vi "Big_LED_control.vi"() -> ()   [LabVIEW 2018]
uses:
  <instrlib>/niDCPower/nidcpower.llb/niDCPower Source Mode.ctl
  <instrlib>/niDCPower/nidcpower.llb/niDCPower Output Function.ctl
  AT lib/AmateurStepperMotor.dll
  <instrlib>/niDMM/nidmm.llb/niDMM Function.ctl
  <instrlib>/niDMM/nidmm.llb/niDMM Resolution in Digits.ctl
  <vilib>/Instr/_visa.llb/VISA Configure Serial Port (Instr).vi
  <instrlib>/niDMM/nidmm.llb/niDMM Configure Measurement Digits.vi
panel:
  out "voltmes_I_LED, V":dbl=-0.00011794146773492402 caption="measurement" format="%_6g"
  out "curmes_I_LED, A":dbl=4.978853713564661e-05 caption="measurement" format="%_6g"
  out "curmes_V_MB, A":dbl=4.978853713564661e-05 caption="measurement" format="%_6g"
  out "voltmes_V_MB, V":dbl=-0.00019003121552656476 caption="measurement" format="%_6g"
  in  "Tab Control 2":enum32{"Шаговик и офир", "Служебная область"}(tab)
  in  "milliseconds to wait":u32=1000
  in  "Go To":dbl
  out "Ophir 1 Char":dbl(graph)=0.02
  in  "DecelerationTime, s":dbl=0.3
  in  "AccelerationTime, s":dbl=0.3
  in  "HoldOn":bool
  in  "Ophir 1 units":string(combo)="1000" caption="Units"
  out "Ophir 1 Over Range":bool caption="Over Range"
  out "Ophir 1 Optical Power":dbl=0.02 caption="Power" format="%#_4g"
  out "Ophir 1 MAX":dbl=0.030000000000000002 caption="MAX" format="%#_5g"
  in  "Ophir 1 Clear":bool caption="Clear"
  in  "StepMultiplicationFactor":dbl=50.0
  in  "StepDivisor":i32(ring)=8 items=["D1"=1, "D2"=2, "D4"=4, "D8"=8, "D16"=16, "D32"=32]
  in  "Speed":dbl=250.0
  in  "Погнали!":bool=TRUE
  in  "Стоп GoTo":bool
  out "Готово":bool
  out "Position":dbl
  in  "Ophir 1 Info":u16(ring)=1 caption="Info" items=["Device : JUNO; s/n:903793", "Head : PD300R-3W   ; s/n:779628"]
  in  "new pos":dbl
  in  "set pos":bool
  out "Device Response":string="*\n"
  in  "Ophir 1 usb channel":i16 caption="usb channel"
  out "Ophir 1 dup Visa Session":refnum<visa-resource-name>="USB0::0x0BD3::0x0777::NI-VISA-60004::RAW" caption="dup Visa Session"
  in  "Ophir 1 Baud Rate (3:9600)":i16(ring)=3 caption="Baud Rate (3:9600)" items=["300", "1200", "4800", "9600", "19200", "38400"]
  out "Ophir 1 Real Optical Power":dbl=2e-05 format="%.6e"
  in  "Ophir 1 GPIB Address (10)":string="10" caption="GPIB Address (10)"
  in  "Ophir 1 Port Number (default 2)":i16=1 caption="Port Number (default 2)" min=0 max=20
  in  "Ophir 1 Select Communication Protocol":u16(ring) caption="Select Communication Protocol" items=["USB", "RS232", "GPIB"]
  out "Ophir 1 error out":errorcluster caption="error out"
  in  "Ophir 1 error in (no error)":errorcluster caption="error in (no error)"
  in  "Ophir 1 Wait":u32=100 caption="Wait"
  out "IsOpen":bool=TRUE
  out "Ophir 1 Initialization":bool=TRUE caption="Initialization"
  in  "Tab Control":T1(tab)
  in  "POWER":bool
  in  "Стоп":bool=TRUE
  in  "Resource Name":refnum<k15>="PXI1Slot2" caption="Источник питания"
  in  "Амперметр":refnum<k15>="PXI1Slot4" caption="NI DMM 1"
  in  "V_MB, V":dbl=2.0 caption="voltage level" format="%_6p"
  in  "curlim_V_MB, A":dbl=0.3 caption="current limit" format="%_6p"
  out "chart_0":dbl(graph)=-0.00019003121552656476 caption="Waveform Chart 5"
  in  "voltlim_I_LED, V":dbl=2.0 caption="current limit" min=0.01 format="%_6p"
  in  "I_LED, A":dbl=0.005 caption="voltage level" format="%_6p"
  out "chart_1":dbl(graph)=-0.00011794146773492402 caption="Waveform Chart 5"
  out "Current Char":dbl(graph)=0.004513189196586609
  in  "Arduino":refnum<visa-resource-name>="COM14"
  in  "Сегменты":bool[](array[boolean])=[FALSE, FALSE, FALSE, FALSE, FALSE, FALSE, FALSE, FALSE, FALSE, FALSE, FALSE, FALSE, FALSE, FALSE, FALSE, FALSE, FALSE, FALSE]
  in  "Вольтметр":refnum<k15>="PXI1Slot5" caption="NI DMM 1"
  out "Voltage Char":dbl(graph)=0.015767553821206093
  in  "Port Name":string="COM4" caption="Порт шаговика"
  in  "wave_lenght":string="600"
  in  "Промер":bool caption="Промер сегмента"
  in  "NI DMM 1 Voltage Range 4":string(combo)="-1" caption="Range"
  in  "NI DMM 1 units 4":string(combo)="1" caption="Units"
  out "Voltage":dbl=0.015767553821206093 format="%_6g"
  in  "NI DMM 1 Current Range 3":string(combo)="1" caption="Range"
  in  "NI DMM 1 units 3":string(combo)="1000" caption="Units"
  out "Current":dbl=0.004513189196586609 format="%_6g"
  out "element":dbl
  out "element 2":dbl
  out "Разряд":dbl
  out "+/-":bool
  out "Power off":bool=TRUE
  in  "Command":string="Cathode"
  in  "Записать":bool
  out "measure output file refnum":refnum<file>
  out "Voltage, V":dbl=0.015767553821206093 caption="Measurement" format="%.5f"
  out "Current, A":dbl=4.513189196586609e-06 caption="Measurement" format="%.5f"
  out "Тип индикатора":string="Cathode"
  out "chart_2":dbl(graph)=-0.000179732680132088
  in  "V_RES, V":dbl caption="voltage level" format="%_6p"
  out "curmes_V_RES, A":dbl=5.996099535583298e-05 caption="measurement" format="%_6g"
  in  "curlim_V_RES, A":dbl=0.1 caption="current limit" min=0.01 format="%_6p"
  in  "measure path":path=path "D:/NI LabVIEW/MultiOpto/MultiOpto_1.2/Logs/SEL"
  out "Enum":enum16{"Exit", "4", "Промер", "2", "1"}(ring)
  out "№ об-ца":dbl=1.0
  out "Темп-ра":dbl=1.0
  out "Сегмент":string
  out "voltmes_V_RES, V":dbl=-0.000179732680132088 caption="measurement" format="%_6g"
  in  "current level range":dbl=0.001 format="%#.6p"
  # "Шаговик"
  # "Офир"
  # "Шаговик"
  # "Офир"
  # "position - это значение абсолютное"
  # "j"
  # "c"
  # "d"
  # "e"
  # "g"
  # "h"
  # "a"
  # "b"
  # "f"
  # "k"
  # "L"
  # "m"
  # "n"
  # "p"
  # "dp"
  # "all"
  # "V_MB 5 В\nогрничение 300 м\n\nV_LED 2,1 В\nограничение 200 м"
  # "единицы мА\nrange 1 А"
  # "1. каждый сегмент включаем по отдельности, резистором постраиваем ток до 10 мА\n2. напряжение V_LED при этом не меняется\n3. в такоом положении промеряем сегменты по отдельности\n4. для промера всего индикатора сразу подстраиваем напряжение при неизменном положении резисторов\n5. ток всех индикаторов = ток одного сегмента (10 мА) * число сегментов (15)\n6. добиваемся этого увеличением V_LED"
  # "единицы В\nrange AUTO"
  # "регклировка суммарного тока через индикатор"
  # "24.063\n\n     I          U\n20 мА  1.3 В\n20 мА  1.4 В\n 7 мА   1.15 В"
  # "24.064\n\n     I          U\n10 мА  2 В\n10 мА  2.15 В\n 7 мА   1.9 В"
  # "автоматизировать подбор напряжения по известному максимальному напряжению и току. ОС по току сегмента"
  # "Р1:  +25°C\nР2:  - 60°C\nР3:  +85°C"
  # "регулировать ток в зависимости от температуры.\nс ростом температуры растет ток.\nпид-регулятор??"
  # "0. ввести номер образца\n1. включить нужный сегмент\n2. ввести его в поле справа\n3. вести температуру в поле слева\n4. нажать кнопку \"промер сегмента\""
  # "\"опрашивать кнопки не чаще, чем раз в секунду. сейчас кликать можно чаще, они загорятся, но ничего не произойдет\""
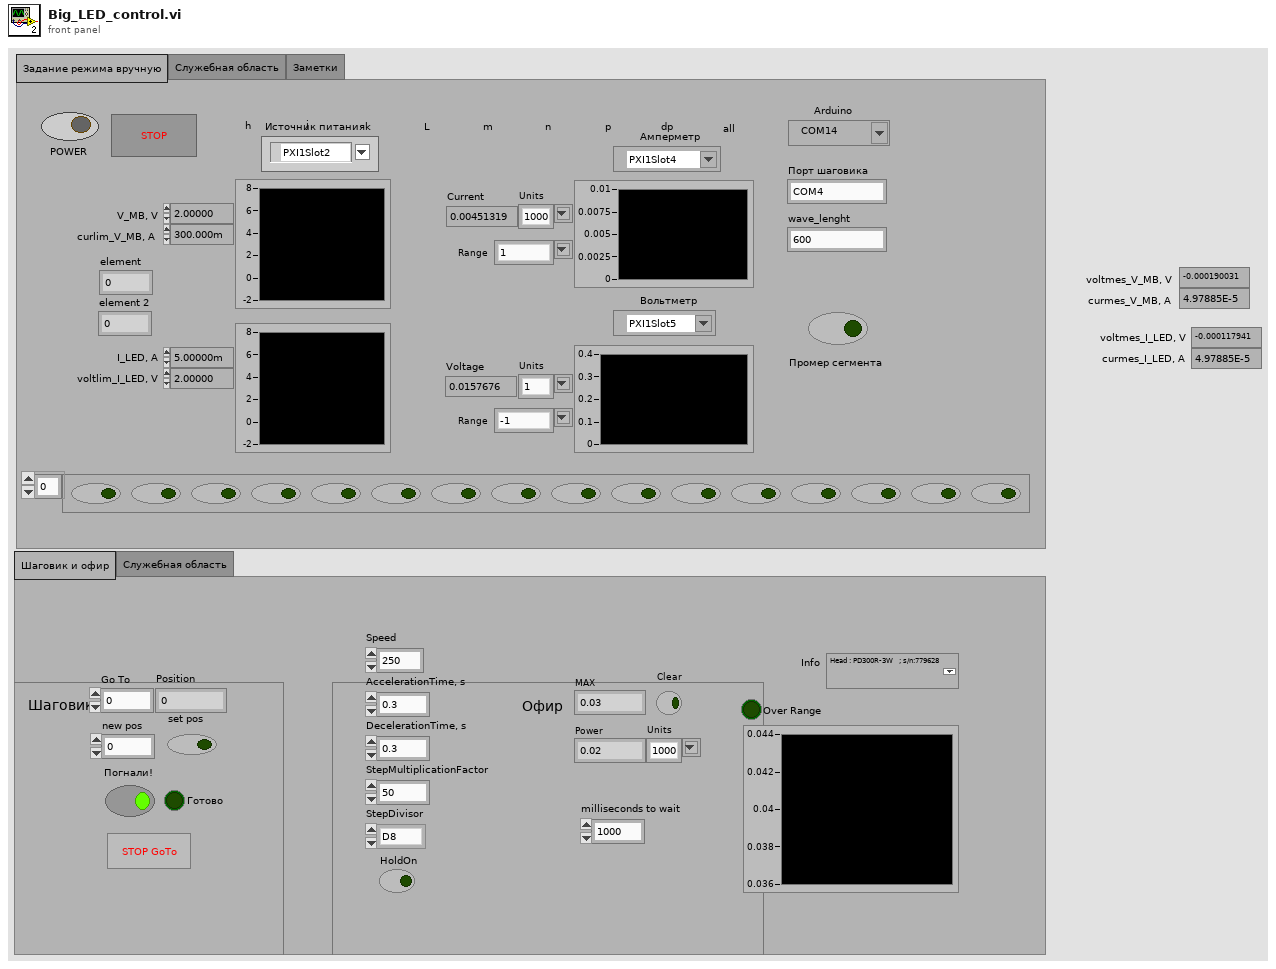
[diagram p1: front panel]
types:
  T1 = enum32{"Задание режима вручную", "Служебная область", "Заметки"}
  T2 = enum16{"open", "replace", "create", "open or create", "replace or create", "replace or create with confirmation"}
  T3 = typedef "niDCPower Output Function.ctl" = i32
  T4 = typedef "niDCPower Source Mode.ctl" = i32
  T5 = typedef "niDMM Function.ctl" = enum16{"DC Volts", "AC Volts", "DC Current", "AC Current", "2-wire Resistance", "4-wire Resistance", "Diode", "Frequency", "Period", "AC Volts DC Coupled", "Capacitance", "Inductance", "Temperature"}
  T6 = typedef "niDMM Resolution in Digits.ctl" = dbl
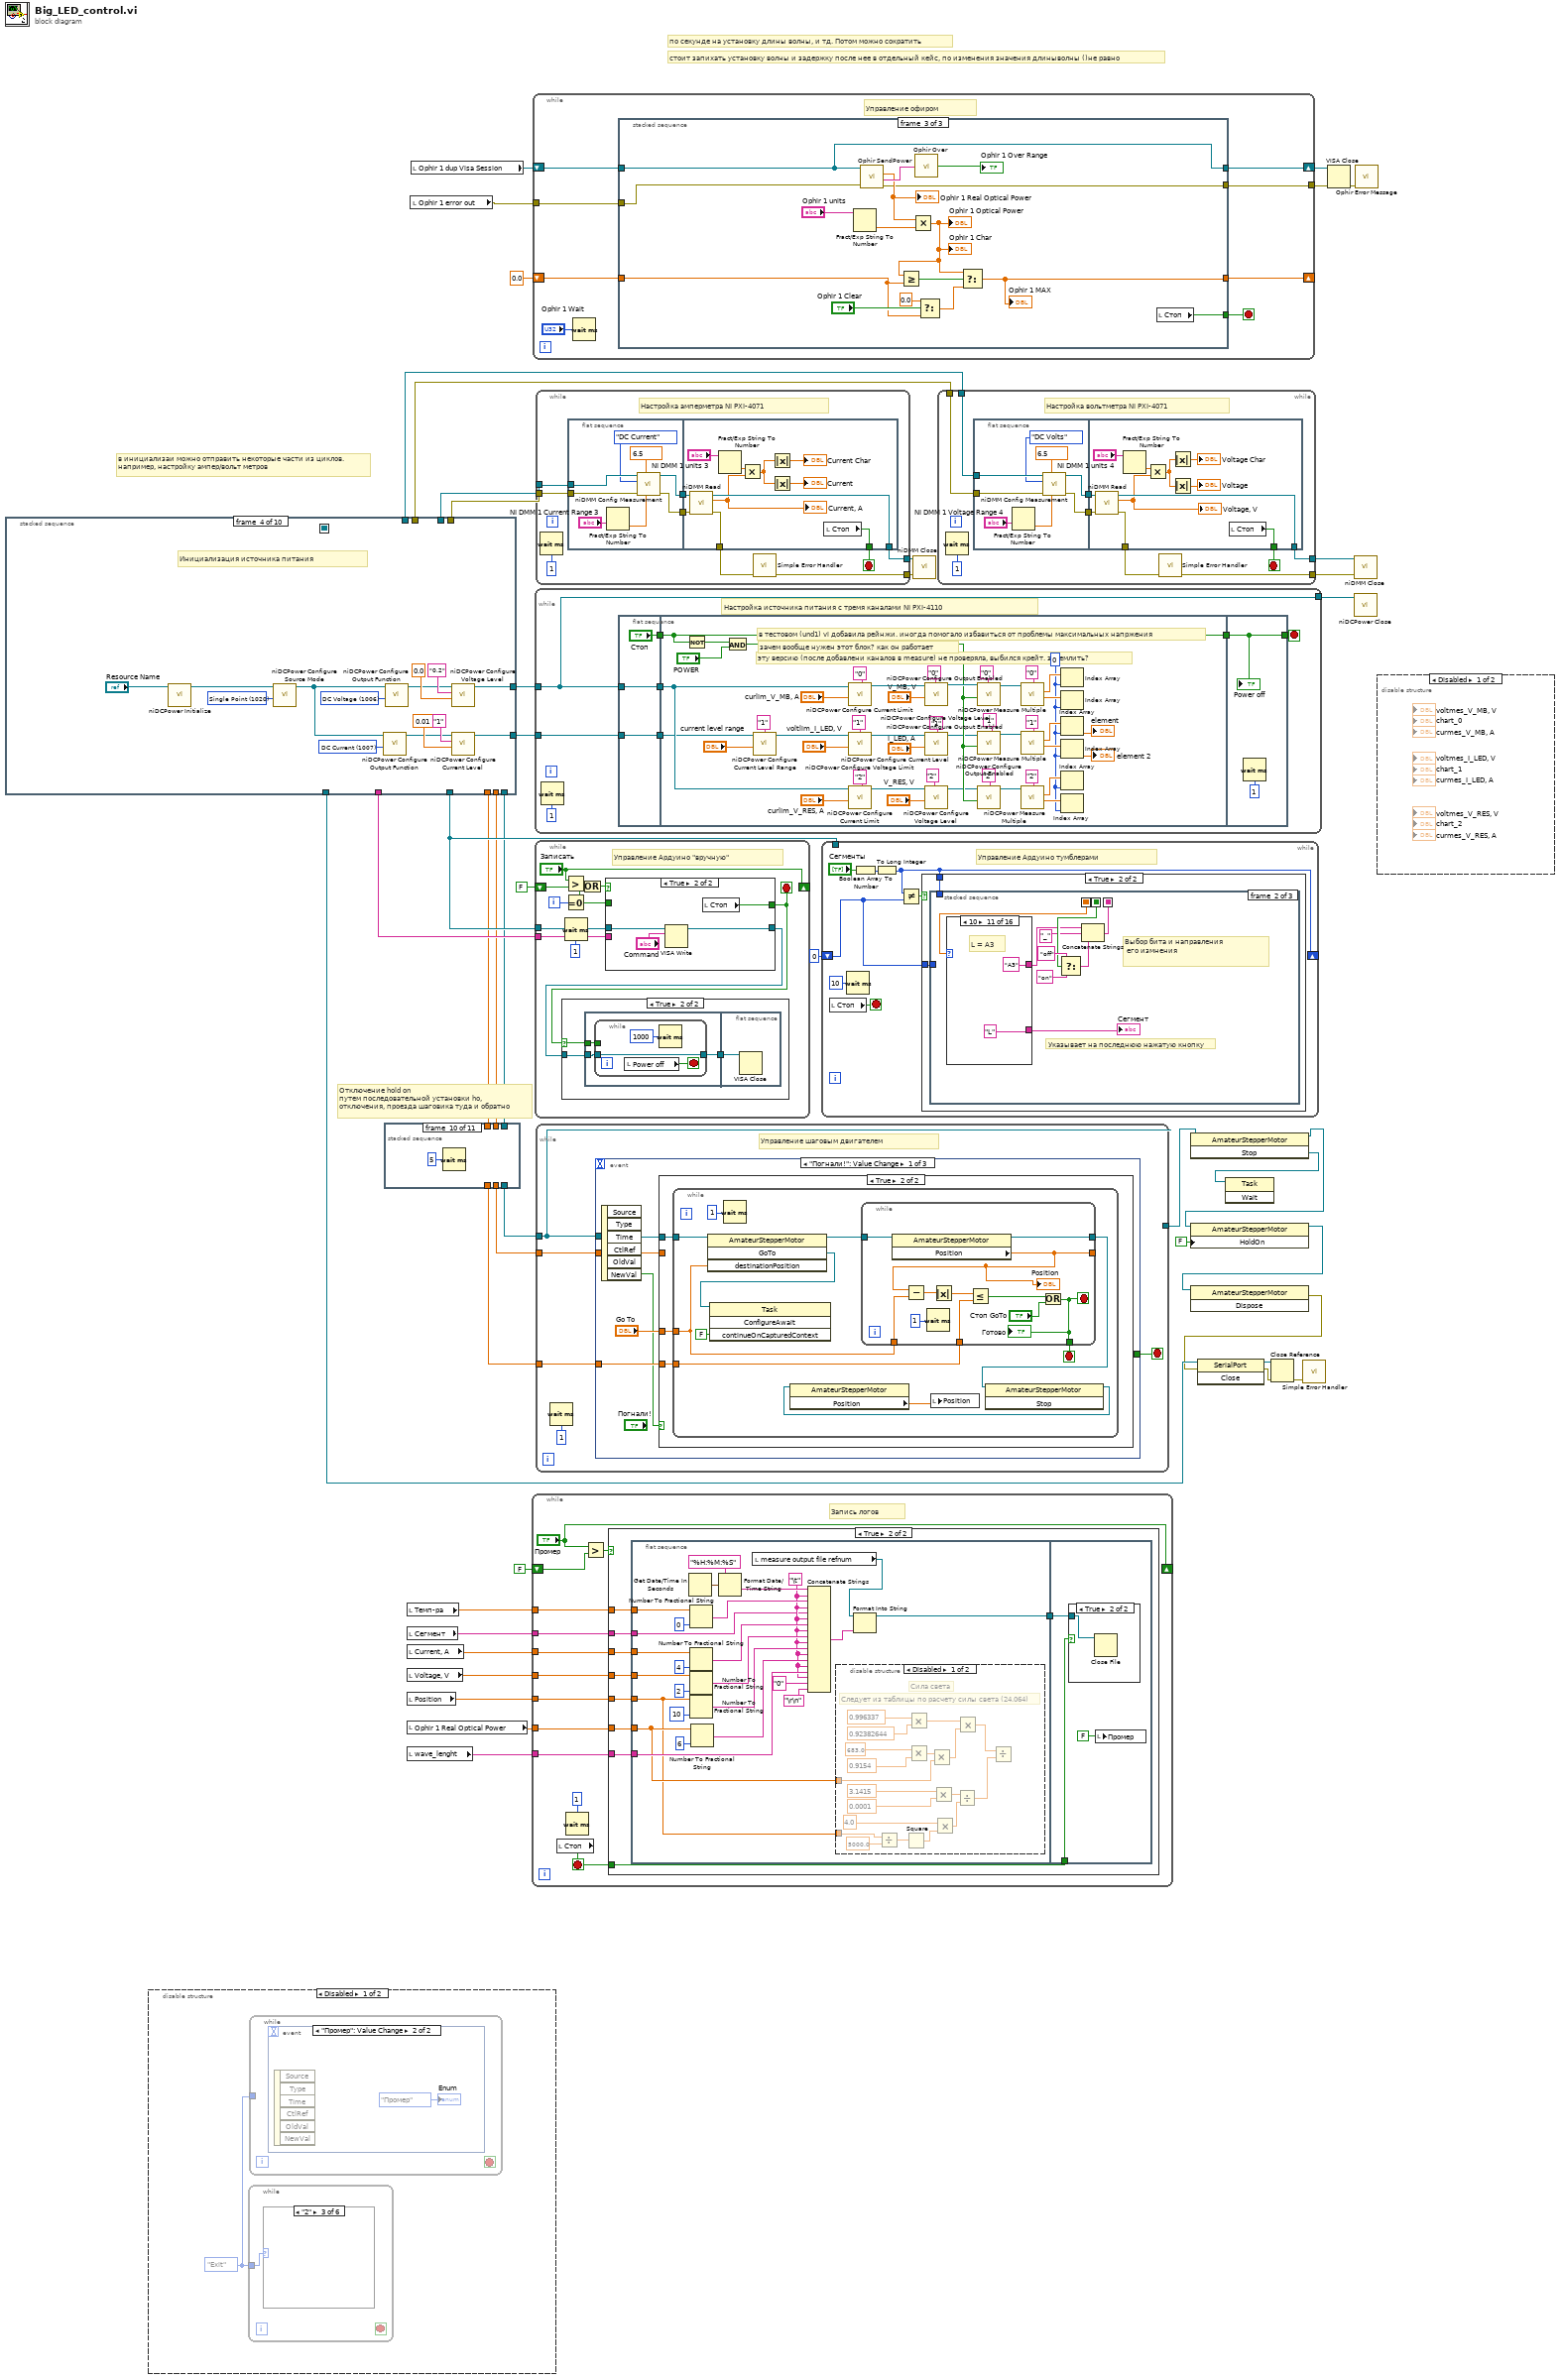
[diagram p0: block diagram]
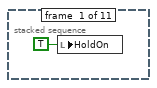
[diagram p3: hidden frame]
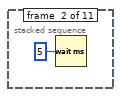
[diagram p4: hidden frame]
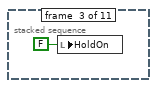
[diagram p5: hidden frame]
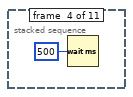
[diagram p6: hidden frame]
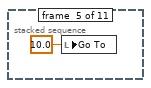
[diagram p7: hidden frame]
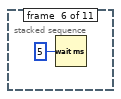
[diagram p8: hidden frame]
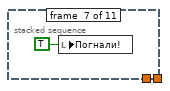
[diagram p9: hidden frame]
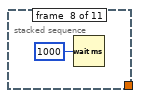
[diagram p10: hidden frame]
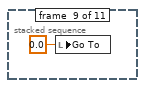
[diagram p11: hidden frame]
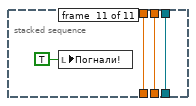
[diagram p12: hidden frame]
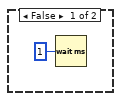
[diagram p13: hidden frame]
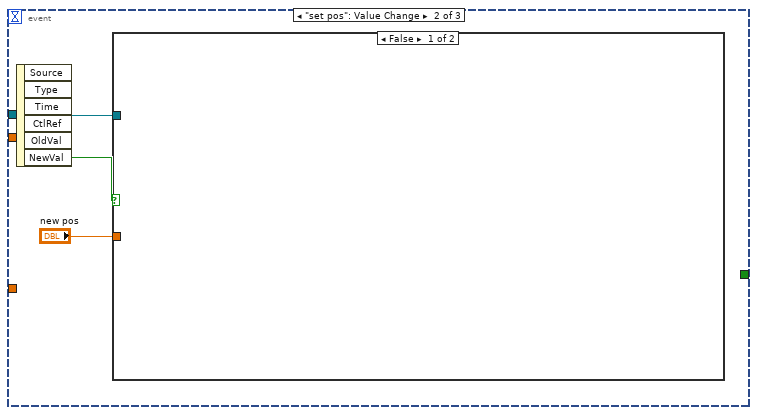
[diagram p14: hidden frame]
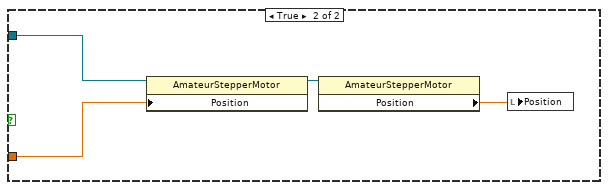
[diagram p15: hidden frame]
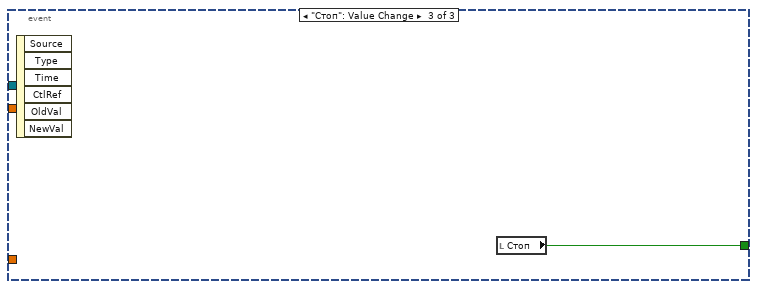
[diagram p16: hidden frame]
diagram:
  # "Отключение hold on\nпутем последовательной установки ho, \nотключения, проезда шаговика туда и обратно"
  # "в инициализаи можно отправить некоторые части из циклов.\nнапример, настройку ампер/вольт метров"
  # "стоит запихать установку волны и задержку после нее в отдельный кейс, по изменения значения длиныволны ()не равно"
  # "по секунде на установку длины волны, и тд. Потом можно сократить"
  n1 = stacked-sequence {
    seq-local: [_ _ _ _ _ _ w108 _ _ _] -> [_ _ _ _ _ _ _ w117 _ _]
    tunnel: [_ _ _ w74 _ _ _ _ _ _] -> w33
    tunnel: [_ w57 _ _ _ _ _ _ _ _] -> w45
    tunnel: [_ w56 _ _ _ _ _ _ _ _] -> w44
    tunnel: [_ _ _ _ w75 _ _ _ _ _] -> w41
    tunnel: [_ _ _ _ _ _ _ _ _ w155] -> w40
    tunnel: [_ _ w60 _ _ _ _ _ _ _] -> w39
    tunnel: [_ _ w59 _ _ _ _ _ _ _] -> w38
    tunnel: [_ _ _ _ _ _ _ w120 _ _] -> w1
    tunnel: [_ _ _ _ _ _ _ w118 _ _] -> w4
    tunnel: [_ _ _ _ _ _ _ w119 _ _] -> w6
    tunnel: [_ _ _ _ _ _ w98 _ _ _] -> w27
    tunnel: [_ _ _ w68 _ _ _ _ _ _] -> w10
    frame #0 {
      w51 = 0.0 ("currentmes_2")
      w52 = FALSE ("Стоп")
      # "ch 1"
      # "Обнуление переменных"
      n2 = local write "POWER"(w52) -> ()
      n3 = local write "Стоп"(w52) -> ()
      n4 = local write "+/-"(w52) -> ()
      n5 = local write "Погнали!"(w52) -> ()
      n6 = local write "Готово"(w52) -> ()
      n7 = local write "Стоп GoTo"(w52) -> ()
      n8 = local write "Speed"(250.0 ("Speed")) -> ()
      n9 = local write "StepMultiplicationFactor"(50.0 ("StepMultiplicationFactor")) -> ()
      n10 = local write "AccelerationTime, s"(0.3 ("AccelerationTime, s")) -> ()
      n11 = local write "DecelerationTime, s"(0.3 ("DecelerationTime, s")) -> ()
      n12 = local write "Go To"(w51) -> ()
      n13 = local write "curmes_V_MB, A"(w51) -> ()
      n14 = local write "curmes_V_RES, A"(w51) -> ()
      n15 = local write "Current"(w51) -> ()
      n16 = local write "Разряд"(w51) -> ()
      n17 = local write "voltmes_I_LED, V"(w51) -> ()
      n18 = local write "Сегменты"(bool[] [FALSE, FALSE, FALSE, FALSE, FALSE, FALSE, FALSE, FALSE, FALSE, FALSE, FALSE, FALSE, FALSE, FALSE, FALSE, FALSE, FALSE, FALSE] ("Сегменты")) -> ()
      n19 = local write "current level range"(0.001 ("current level range")) -> ()
      n20 = local write "Command"("zero" ("Command 2")) -> ()
    }
    frame #1 {
      # "Инициализация амперметра"
      n21 = call <instrlib>:"niDMM Initialize.vi"("Instrument Descriptor"="Амперметр") -> ("error out"=w57:errorcluster, "instrument handle out"=w56:refnum<k15>)  [unwired: 9 in]
    }
    frame #2 {
      # "Инициализация вольтметра"
      n22 = call <instrlib>:"niDMM Initialize.vi"("Instrument Descriptor"="Вольтметр") -> ("error out"=w59:errorcluster, "instrument handle out"=w60:refnum<k15>)  [unwired: 9 in]
    }
    frame #3 {
      w61 = T3 1007 items=["DC Voltage"=1006, "DC Current"=1007, "Pulse Voltage"=1049, "Pulse Current"=1050] ("output function")
      w62 = T3 1006 items=["DC Voltage"=1006, "DC Current"=1007, "Pulse Voltage"=1049, "Pulse Current"=1050] ("output function")
      w66 = T4 1020 items=["Single Point"=1020, "Sequence"=1021] ("source mode")
      # "Инициализация источника питания"
      n23 = call <instrlib>:"niDCPower Initialize.vi"("resource name"="Resource Name") -> ("instrument handle out"=w67:refnum<k15>)  [unwired: 3 in, 7 out]
      n24 = call <instrlib>:"niDCPower Configure Source Mode.vi"("source mode"=w66, "instrument handle"=w67) -> ("instrument handle out"=w65:refnum<k15>)  [unwired: 1 in, 8 out]
      n25 = call <instrlib>:"niDCPower Configure Output Function.vi"("output function"=w61, "instrument handle"=w65) -> ("instrument handle out"=w63:refnum<k15>)  [unwired: 8 in, 1 out]
      n26 = call <instrlib>:"niDCPower Configure Output Function.vi"("output function"=w62, "instrument handle"=w65) -> ("instrument handle out"=w64:refnum<k15>)  [unwired: 8 in, 1 out]
      n27 = call <instrlib>:"niDCPower Configure Voltage Level.vi"("voltage level"=0.0, "channel name"="0,2", "instrument handle"=w64) -> ("instrument handle out"=w74:refnum<k15>)  [unwired: 7 in, 1 out]
      n28 = call <instrlib>:"niDCPower Configure Current Level.vi"("current level"=0.01, "channel name"="1", "instrument handle"=w63) -> ("instrument handle out"=w68:refnum<k15>)  [unwired: 7 in, 1 out]
    }
    frame #4 {
      # "Инициализация Ардуино"
      n29 = call-poly "VISA Configure Serial Port"("VISA resource name"="Arduino", "baud rate (9600)"=u32 9600) -> ("VISA resource name out"=w75:refnum<visa-resource-name>)  [unwired: 12 in, 1 out]
    }
    frame #5 {
      # "Инициализация офира"
      n30 = call "Ophir InitCom.vi"("GPIB Address (default 10)"="Ophir 1 GPIB Address (10)", "Communication (default USB 0)"="Ophir 1 Select Communication Protocol", "USB Channel number (default 0)"="Ophir 1 usb channel", "Port Number (default 2)"="Ophir 1 Port Number (default 2)", "error in (no error)"="Ophir 1 error in (no error)", "Baud Rate (3:9600)"="Ophir 1 Baud Rate (3:9600)") -> ("dup Visa Session"=w84:refnum<visa-resource-name>, "error out"=w83:errorcluster)  [unwired: 1 out]
      n31 = call "Ophir InstrInfo.vi"("Visa Session"=w84, "error in (no error)"=w83) -> ("dup Visa Session"=w96:refnum<visa-resource-name>, "Instrument Info"=w78:string, "error out"=w94:errorcluster)
      n32 = call "Ophir HeadInfo.vi"("Visa Session"=w96, "error in (no error)"=w94) -> ("error out"=w93:errorcluster, "dup Visa Session"=w95:refnum<visa-resource-name>, "Head Info"=w92:string)  [unwired: 6 out]
      n33 = call "Ophir InfoStrings.vi"("error in (no error)"=w93, "Head Info"=w92, "Instrument Info"=w78) -> ("error out"=w91:errorcluster, "Strings Array"=w90:string[])
      n34 = property on="Ophir 1 Info" class="Ring (strict)"("Strings []"=w90) -> ()  [unwired: 2 in, 2 out]
      n35 = call "Ophir ConfigDevice.vi"("Visa Session"=w95, "Measure Choice (0:Power)"=u16 0, "error in (no error)"=w91) -> ("dup Visa Session"=→"Ophir 1 dup Visa Session":refnum<visa-resource-name>, "OK ?"=→"Ophir 1 Initialization":bool, "error out"=→"Ophir 1 error out":errorcluster)  [unwired: 1 out]
    }
    frame #6 {
      w102 = 100 ("WriteTimeout")
      w107 = 1 items=["None", "One", "Two", "OnePointFive"] ("stopBits")
      w104 = 0 items=["None", "Odd", "Even", "Mark", "Space"] ("parity")
      # "убрали открытие порта. шаговик его и так сам откроет"
      # "Инициализация шаговика ч.1"
      n36 = constructor class="SerialPort"("portName"="Port Name", "baudRate"=57600, "parity"=w104, "dataBits"=8, "stopBits"=w107) -> (reference out=w101:refnum<k24>, error out=w100:errorcluster)  [unwired: 3 in, 6 out]
      n37 = property class="SerialPort"(reference=w101, error in=w100, "WriteTimeout"=w102, "ReadTimeout"=w102) -> (reference out=w98:refnum<k24>)  [unwired: 1 out]
      n38 = constructor class="AmateurStepperMotor"("serialPort"=w98) -> (reference out=w108:refnum<k24>, error out=w99:errorcluster)  [unwired: 3 in, 2 out]
      n39 = flat-sequence {
        tunnel: w99 -> [_]
        tunnel: w98 -> [w110]
        frame #0 {
          n40 = property class="SerialPort"(reference=w110) -> ("IsOpen"=→"IsOpen":bool)  [unwired: 1 in, 2 out]
        }
      }
    }
    frame #7 {
      # "стоит допустить изменение\nтих параметров в цикле, а не только \nпри инициализации"
      # "это те самые 50 шагов за мм"
      # "Инициализация шаговика ч.2"
      n41 = property class="AmateurStepperMotor"(reference=w117, "Speed"="Speed", "StepDivisor"="StepDivisor", "StepMultiplicationFactor"="StepMultiplicationFactor", "AccelerationTime"="AccelerationTime, s", "DecelerationTime"="DecelerationTime, s", "HoldOn"="HoldOn") -> (reference out=w120:refnum<k24>, "Position"=w118:dbl, "PositioningPrecision"=w119:dbl)  [unwired: 1 in, 1 out]
    }
    frame #8 {
      w126 = "\t"
      # "Инициализация логов"
      n42 = local read "№ об-ца"() -> (w122:dbl)
      n43 = Number To Fractional String(number=w122, precision (6)=i16 0) -> (F-format string=w123:string)  [unwired: 2 in]
      n44 = Get Date/Time In Seconds() -> (seconds since 1Jan1904=w144:timestamp)
      n45 = Build Path(base path="measure path", name or relative path=w123) -> (appended path=w140:path)
      n46 = call <vilib>:"Check if File or Folder Exists.vi"("path"=w140) -> ("file or folder exists?"=w141:bool, "dup path"=w142:path)  [unwired: 8 in, 1 out]
      n47 = Format Date/Time String(time format string (%c)="MES %d %m %y %H.%M.%S", seconds (now)=w144) -> (date/time string=w145:string)  [unwired: 1 in]
      n48 = case shown="False" w141 {
        tunnel: w142 -> [w153 w154]
        tunnel: [w152 w154] -> w143
        frame False {
          n49 = Create Folder(path (use dialog)=w153) -> (created path=w152:path)  [unwired: 2 in, 2 out]
        }
        frame True {
        }
      }
      n50 = Concatenate Strings(w145, ".xls" ("string")) -> (w146:string)
      n51 = Build Path(base path=w143, name or relative path=w146) -> (appended path=w147:path)
      n52 = Open/Create/Replace File(file path (use dialog)=w147, operation (0:open)=T2."open or create", access (0:read/write)=enum16{"read/write", "read-only", "write-only"}."read/write") -> (refnum out=w148:refnum<file>)  [unwired: 3 in, 2 out]
      n53 = Set File Position(refnum=w148, from (0:start)=enum16{"start", "end", "current"}."end") -> (refnum out=w150:refnum<file>)  [unwired: 2 in, 1 out]
      n54 = Format Into String(initial string=w150, "Time" ("string"), w126, "Temperature, C" ("string"), w126, "Segment" ("string"), w126, "Current, mA" ("string"), w126, "Voltage, V" ("input 7"), w126, "Distance, m" ("string"), w126, "Power, W " ("string"), w126, "Wavelenght, nm" ("input 17"), w126, "Candlepower, kd" ("string"), "\r\n") -> (resulting string=→"measure output file refnum":refnum<file>)  [unwired: 2 in, 1 out]
    }
    frame #9 {
      # "Begin VI: ОК или ОА?"
      n55 = disable-structure shown="Disabled" {
        disable-tunnel: [w158 _] -> w155
        frame Disabled {
          n56 = call "Begin.vi"() -> ("Темп-ра"=→"Темп-ра":dbl, "№ об-ца"=→"№ об-ца":dbl, "String"=w158:string)  [unwired: 6 in]
          "Тип индикатора" <- w158
          n57 = local write "Command"(w158) -> ()
        }
        frame Enabled {
        }
      }
    }
  }
  n58 = disable-structure shown="Disabled" {
    frame Disabled {
      w159 = enum16{"Exit", "4", "Промер", "2", "1"}."Exit"
      n59 = while {
        tunnel: w159 -> [w160]
        stop <- _ stop-if-true
        n60 = case shown="\"2\"" w160 {
          frame "Exit", Default {
          }
          frame "4" {
          }
          frame "2" {
          }
          frame "2" {
          }
          frame "1" {
          }
          frame "Промер" {
          }
        }
      }
      n61 = while {
        tunnel: w159 -> [_]
        stop <- _ stop-if-true
        n62 = event shown="[1] \"Промер\": Value Change" {
          selector: _ -> [_ _]
          dyn-events: _ -> [_ _]
          timeout: _ -> [_ _]
          event Timeout {
            n63 = event-data() -> ()  [unwired: 1 in, 3 out]
          }
          event "Промер": Value Change {
            n64 = event-data() -> ()  [unwired: 1 in, 6 out]
            "Enum" <- enum16{"Exit", "4", "Промер", "2", "1"}."Промер" ("Enum")
          }
        }
      }
    }
    frame Enabled {
    }
  }
  n65 = stacked-sequence {
    tunnel: w6 -> [_ _ _ _ _ _ _ _ _ _ w174]
    tunnel: [_ _ _ _ _ _ _ _ _ _ w174] -> w5
    tunnel: w4 -> [_ _ _ _ _ _ _ _ _ _ w173]
    tunnel: [_ _ _ _ _ _ _ _ _ _ w173] -> w3
    tunnel: [_ _ _ _ _ _ _ _ _ _ w172] -> w2
    tunnel: w1 -> [_ _ _ _ _ _ _ _ _ _ w172]
    frame #0 {
      n66 = local write "HoldOn"(TRUE ("HoldOn")) -> ()
    }
    frame #1 {
      n67 = Wait (ms)(milliseconds to wait=u32 5) -> ()  [unwired: 1 out]
    }
    frame #2 {
      n68 = local write "HoldOn"(FALSE ("HoldOn")) -> ()
    }
    frame #3 {
      n69 = Wait (ms)(milliseconds to wait=u32 500) -> ()  [unwired: 1 out]
    }
    frame #4 {
      n70 = local write "Go To"(10.0 ("Go To")) -> ()
    }
    frame #5 {
      n71 = Wait (ms)(milliseconds to wait=u32 5) -> ()  [unwired: 1 out]
    }
    frame #6 {
      n72 = local write "Погнали!"(TRUE ("Погнали!")) -> ()
    }
    frame #7 {
      n73 = Wait (ms)(milliseconds to wait=u32 1000) -> ()  [unwired: 1 out]
    }
    frame #8 {
      n74 = local write "Go To"(0.0 ("Go To")) -> ()
    }
    frame #9 {
      n75 = Wait (ms)(milliseconds to wait=u32 5) -> ()  [unwired: 1 out]
    }
    frame #10 {
      n76 = local write "Погнали!"(TRUE ("Погнали!")) -> ()
    }
  }
  n77 = local read "Темп-ра"() -> (w8:dbl)
  n78 = local read "Сегмент"() -> (w7:string)
  n79 = local read "Current, A"() -> (w26:dbl)
  n80 = local read "Voltage, V"() -> (w25:dbl)
  n81 = local read "Position"() -> (w24:dbl)
  n82 = local read "Ophir 1 Real Optical Power"() -> (w23:dbl)
  n83 = local read "wave_lenght"() -> (w22:string)
  n84 = local read "Ophir 1 error out"() -> (w31:errorcluster)
  n85 = local read "Ophir 1 dup Visa Session"() -> (w32:refnum<visa-resource-name>)
  n86 = while {
    tunnel: w26 -> [w187]
    tunnel: w25 -> [w186]
    tunnel: w24 -> [w185]
    tunnel: w23 -> [w184]
    tunnel: w22 -> [w183]
    shift-right: ["Промер"] -> _
    shift-left: FALSE ("Промер сегмента") -> [w180]
    tunnel: w8 -> [w177]
    tunnel: w7 -> [w176]
    stop <- w178 stop-if-true
    # "Запиcь логов"
    n87 = local read "Стоп"() -> (w178:bool)
    n88 = Wait (ms)(milliseconds to wait=u32 1) -> ()  [unwired: 1 out]
    n89 = Greater?(x="Промер", y=w180) -> (0:w181:bool)
    n90 = case shown="True" w181 {
      tunnel: w187 -> [_ w196]
      tunnel: w186 -> [_ w195]
      tunnel: w185 -> [_ w192]
      tunnel: w184 -> [_ w193]
      tunnel: w183 -> [_ w194]
      tunnel: w178 -> [_ w190]
      tunnel: w177 -> [_ w189]
      tunnel: w176 -> [_ w188]
      frame False {
      }
      frame True {
        n91 = flat-sequence {
          tunnel: w196 -> [w214]
          tunnel: w195 -> [w213]
          tunnel: w194 -> [w211]
          tunnel: w193 -> [w210]
          tunnel: w192 -> [w209]
          tunnel: [w204] -> w191
          tunnel: w189 -> [w203]
          tunnel: w188 -> [w197]
          tunnel: w191 -> [w244]
          tunnel: w190 -> [w243]
          frame #0 {
            w199 = "\t"
            n92 = Get Date/Time In Seconds() -> (seconds since 1Jan1904=w222:timestamp)
            n93 = Number To Fractional String(number=w203, precision (6)=i16 0) -> (F-format string=w201:string)  [unwired: 2 in]
            n94 = Number To Fractional String(number=w214, precision (6)=i16 4) -> (F-format string=w217:string)  [unwired: 2 in]
            n95 = Number To Fractional String(number=w213, precision (6)=i16 2) -> (F-format string=w216:string)  [unwired: 2 in]
            n96 = Number To Fractional String(number=w209, precision (6)=i16 10) -> (F-format string=w215:string)  [unwired: 2 in]
            n97 = Number To Fractional String(number=w210, precision (6)=i16 6) -> (F-format string=w212:string)  [unwired: 2 in]
            n98 = Format Date/Time String(time format string (%c)="%H:%M:%S", seconds (now)=w222) -> (date/time string=w220:string)  [unwired: 1 in]
            n99 = local read "measure output file refnum"() -> (w218:refnum<file>)
            n100 = Concatenate Strings(w220, w199, w201, w199, w197, w199, w217, w199, w216, w199, w215, w199, w212, w199, w211, w199, "0" ("string"), "\r\n") -> (w219:string)
            n101 = disable-structure shown="Disabled" {
              disable-tunnel: w210 -> [w234 _]
              disable-tunnel: w209 -> [w224 _]
              frame Disabled {
                # "Сила света"
                # "Следует из таблицы по расчету силы света (24.064)"
                n102 = Divide(x=w224, y=5000.0) -> (x/y=w226:dbl)
                n103 = Square(x=w226) -> (x^2=w225:dbl)
                n104 = Multiply(x=0.996337, y=0.92382644) -> (x*y=w239:dbl)
                n105 = Multiply(x=683.0, y=0.9154) -> (x*y=w235:dbl)
                n106 = Multiply(x=w235, y=w234) -> (x*y=w233:dbl)
                n107 = Multiply(x=3.1415, y=0.0001) -> (x*y=w229:dbl)
                n108 = Multiply(x=4.0, y=w225) -> (x*y=w228:dbl)
                n109 = Divide(x=w229, y=w228) -> (x/y=w230:dbl)
                n110 = Multiply(x=w239, y=w233) -> (x*y=w238:dbl)
                n111 = Divide(x=w238, y=w230) -> ()  [unwired: 1 out]
              }
              frame Enabled {
              }
            }
            n112 = Format Into String(initial string=w218, w219) -> (resulting string=w204:refnum<file>)  [unwired: 2 in, 1 out]
          }
          frame #1 {
            n113 = case shown="True" w243 {
              tunnel: w244 -> [_ w245]
              frame False {
              }
              frame True {
                n114 = Close File(refnum=w245) -> ()  [unwired: 1 in, 2 out]
              }
            }
            n115 = local write "Промер"(FALSE ("Промер")) -> ()
          }
        }
      }
    }
  }
  n116 = while {
    tunnel: w31 -> [w252]
    shift-right: [w248] -> _
    shift-left: 0.0 ("t") -> [w251]
    shift-right: [w249] -> w20
    shift-left: w32 -> [w253]
    tunnel: [w247] -> w19
    stop <- w246 stop-if-true
    # "Управление офиром"
    n117 = Wait (ms)(milliseconds to wait="Ophir 1 Wait") -> ()  [unwired: 1 out]
    n118 = stacked-sequence {
      tunnel: w253 -> [w257 _ w260]
      tunnel: w252 -> [w256 _ w262]
      tunnel: w251 -> [_ _ w263]
      tunnel: [_ _ w260] -> w249
      tunnel: [_ _ w264] -> w248
      tunnel: [_ _ w261] -> w247
      tunnel: [_ _ w259] -> w246
      frame #0 {
        n119 = call "light_setWaveLenght.vi"("error in (no error)"=w256, "Visa Session"=w257, "wave_lenght"="wave_lenght") -> ("Device Response"=→"Device Response":string)  [unwired: 6 in, 2 out]
      }
      frame #1 {
        n120 = Wait (ms)(milliseconds to wait="milliseconds to wait") -> ()  [unwired: 1 out]
      }
      frame #2 {
        n121 = Fract/Exp String To Number(string="Ophir 1 units") -> (number=w267:dbl)  [unwired: 3 in, 1 out]
        n122 = call "Ophir SendPower.vi"("Visa Session"=w260, "error in (no error)"=w262) -> ("Value Number"=w266:dbl, "Value String"=w273:string, "error out"=w261:errorcluster)  [unwired: 1 out]
        "Ophir 1 Real Optical Power" <- w266
        n123 = Multiply(x=w266, y=w267) -> (x*y=w270:dbl)
        "Ophir 1 Char" <- w270
        "Ophir 1 Optical Power" <- w270
        n124 = Greater Or Equal?(x=w270, y=w263) -> (x >= y?=w271:bool)
        n125 = call "Ophir Over.vi"("Value String"=w273) -> ("Overrange"=→"Ophir 1 Over Range":bool)
        n126 = Select(t=0.0, s="Ophir 1 Clear", f=w263) -> (s? t:f=w269:dbl)
        n127 = Select(t=w270, s=w271, f=w269) -> (s? t:f=w264:dbl)
        "Ophir 1 MAX" <- w264
        n128 = local read "Стоп"() -> (w259:bool)
      }
    }
  }
  n129 = while {
    tunnel: w33 -> [w279]
    tunnel: [w279] -> w42
    tunnel: w10 -> [w276]
    stop <- w275 stop-if-true
    # "Настройка источника питания с тремя каналами NI PXI-4110"
    n130 = Wait (ms)(milliseconds to wait=u32 1) -> ()  [unwired: 1 out]
    n131 = flat-sequence {
      tunnel: w279 -> [w285]
      tunnel: [w285] -> w281
      tunnel: ["Стоп"] -> w280
      tunnel: [w283] -> w277
      tunnel: w276 -> [w283]
      tunnel: w281 -> [w326]
      tunnel: w280 -> [w330]
      tunnel: [w330] -> w278
      tunnel: w277 -> [w294]
      tunnel: [w332] -> w275
      tunnel: w278 -> [w332]
      frame #0 {
      }
      frame #1 {
        w295 = 0 ("index")
        # "эту версию (после добавлени каналов в measure) не проверяла, выбился крейт. заземлить?"
        # "зачем вообще нужен этот блок? как он работает"
        # "в тестовом (und1) vi добавила рейнжи. иногда помогало избавиться от проблемы максимальных напржения"
        n132 = Not(x=w330) -> (.not. x?=w329:bool)
        n133 = And(x=w329, y="POWER") -> (x .and. y?=w325:bool)
        n134 = call <instrlib>:"niDCPower Configure Current Level Range.vi"("current level range"="current level range", "channel name"="1", "instrument handle"=w294) -> ("instrument handle out"=w293:refnum<k15>)  [unwired: 7 in, 1 out]
        n135 = call <instrlib>:"niDCPower Configure Current Limit.vi"("current limit"="curlim_V_MB, A", "channel name"="0", "instrument handle"=w326) -> ("instrument handle out"=w316:refnum<k15>)  [unwired: 7 in, 1 out]
        n136 = call <instrlib>:"niDCPower Configure Voltage Limit.vi"("voltage limit"="voltlim_I_LED, V", "channel name"="1", "instrument handle"=w293) -> ("instrument handle out"=w320:refnum<k15>)  [unwired: 7 in, 1 out]
        n137 = call <instrlib>:"niDCPower Configure Current Limit.vi"("current limit"="curlim_V_RES, A", "channel name"="2", "instrument handle"=w326) -> ("instrument handle out"=w310:refnum<k15>)  [unwired: 7 in, 1 out]
        n138 = call <instrlib>:"niDCPower Configure Voltage Level.vi"("voltage level"="V_MB, V", "channel name"="0", "instrument handle"=w316) -> ("instrument handle out"=w327:refnum<k15>)  [unwired: 7 in, 1 out]
        n139 = call <instrlib>:"niDCPower Configure Current Level.vi"("current level"="I_LED, A", "channel name"="1", "instrument handle"=w320) -> ("instrument handle out"=w321:refnum<k15>)  [unwired: 7 in, 1 out]
        n140 = call <instrlib>:"niDCPower Configure Voltage Level.vi"("voltage level"="V_RES, V", "channel name"="2", "instrument handle"=w310) -> ("instrument handle out"=w311:refnum<k15>)  [unwired: 7 in, 1 out]
        n141 = call <instrlib>:"niDCPower Configure Output Enabled.vi"("output enabled"=w325, "channel name"="0", "instrument handle"=w327) -> ("instrument handle out"=w304:refnum<k15>)  [unwired: 7 in, 1 out]
        n142 = call <instrlib>:"niDCPower Configure Output Enabled.vi"("output enabled"=w325, "channel name"="1", "instrument handle"=w321) -> ("instrument handle out"=w297:refnum<k15>)  [unwired: 7 in, 1 out]
        n143 = call <instrlib>:"niDCPower Configure Output Enabled.vi"("output enabled"=w325, "channel name"="2", "instrument handle"=w311) -> ("instrument handle out"=w296:refnum<k15>)  [unwired: 7 in, 1 out]
        n144 = call <instrlib>:"niDCPower Measure Multiple.vi"("channel name"="0", "instrument handle"=w304) -> ("current measurements"=w302:dbl[], "voltage measurements"=w303:dbl[])  [unwired: 6 in, 2 out]
        n145 = call <instrlib>:"niDCPower Measure Multiple.vi"("channel name"="1", "instrument handle"=w297) -> ("current measurements"=w300:dbl[], "voltage measurements"=w301:dbl[])  [unwired: 6 in, 2 out]
        n146 = call <instrlib>:"niDCPower Measure Multiple.vi"("channel name"="2", "instrument handle"=w296) -> ("current measurements"=w298:dbl[], "voltage measurements"=w299:dbl[])  [unwired: 6 in, 2 out]
        n147 = Index Array(array=w303, index=w295) -> ()  [unwired: 1 out]
        n148 = Index Array(array=w302, index=w295) -> ()  [unwired: 1 out]
        n149 = Index Array(array=w301, index=w295) -> (element=→"element":dbl)
        n150 = Index Array(array=w300, index=w295) -> (element=→"element 2":dbl)
        n151 = Index Array(array=w299, index=w295) -> ()  [unwired: 1 out]
        n152 = Index Array(array=w298, index=w295) -> ()  [unwired: 1 out]
      }
      frame #2 {
        n153 = Wait (ms)(milliseconds to wait=u32 1) -> ()  [unwired: 1 out]
        "Power off" <- w332
      }
    }
  }
  n154 = while {
    tunnel: w41 -> [w340]
    shift-right: ["Записать"] -> _
    shift-left: FALSE ("Записать") -> [w342]
    tunnel: w40 -> [w338]
    i -> [w339]
    stop <- w333 stop-if-true
    # "Управление Ардуино \"вручную\""
    n155 = Greater?(x="Записать", y=w342) -> (0:w336:bool)
    n156 = Equal To 0?(x=w339) -> (x = 0?=w335:bool)
    n157 = Wait (ms)(milliseconds to wait=u32 1) -> ()  [unwired: 1 out]
    n158 = Or(x=w336, y=w335) -> (x .or. y?=w337:bool)
    n159 = case shown="True" w337 {
      tunnel: w340 -> [w354 w359]
      tunnel: [w355 w358] -> w333
      tunnel: w338 -> [_ _]
      tunnel: w335 -> [_ _]
      tunnel: [w354 w356] -> w334
      frame False {
        n160 = local read "Стоп"() -> (w355:bool)
      }
      frame True {
        n161 = VISA Write(VISA resource name=w359, write buffer="Command") -> (VISA resource name out=w356:refnum<visa-resource-name>)  [unwired: 1 in, 2 out]
        n162 = local read "Стоп"() -> (w358:bool)
      }
    }
    n163 = case shown="True" w333 {
      selector: w333 -> [_ w344]
      tunnel: w334 -> [_ w346]
      frame False {
      }
      frame True {
        n164 = flat-sequence {
          tunnel: w346 -> [w349]
          tunnel: [w348] -> w345
          tunnel: w344 -> [w347]
          tunnel: w345 -> [w353]
          frame #0 {
            n165 = while {
              tunnel: w349 -> [w352]
              tunnel: [w352] -> w348
              tunnel: w347 -> [_]
              stop <- w350 stop-if-true
              n166 = local read "Power off"() -> (w350:bool)
              n167 = Wait (ms)(milliseconds to wait=u32 1000) -> ()  [unwired: 1 out]
            }
          }
          frame #1 {
            n168 = VISA Close(VISA resource name=w353) -> ()  [unwired: 1 in, 1 out]
          }
        }
      }
    }
  }
  n169 = while {
    tunnel: [w366] -> w34
    tunnel: w44 -> [w364]
    tunnel: w45 -> [w363]
    tunnel: [w360] -> w35
    stop <- w362 stop-if-true
    # "Настройка амперметра NI PXI-4071"
    n170 = Wait (ms)(milliseconds to wait=u32 1) -> ()  [unwired: 1 out]
    n171 = flat-sequence {
      tunnel: [w373] -> w368
      tunnel: w364 -> [w371]
      tunnel: w363 -> [w375]
      tunnel: [w372] -> w367
      tunnel: w368 -> [w384]
      tunnel: w367 -> [w387]
      tunnel: [w383] -> w362
      tunnel: [w382] -> w360
      tunnel: [w381] -> w361
      frame #0 {
        w369 = T6 6.5 items=["3 1/2"=3.5, "4 1/2"=4.5, "5 1/2"=5.5, "6 1/2"=6.5, "7 1/2"=7.5] ("Resolution in Digits")
        n172 = Fract/Exp String To Number(string="NI DMM 1 Current Range 3") -> (number=w374:dbl)  [unwired: 3 in, 1 out]
        n173 = call-poly <instrlib>:"niDMM Config Measurement.vi"("Range"=w374, "Resolution in Digits"=w369, "error in (no error)"=w375, "Function"=niDMM_Function."DC Current" ("Measurement Type"), "instrument handle"=w371) -> ("error out"=w372:errorcluster, "instrument handle out"=w373:refnum<k15>)  [unwired: 5 in]
      }
      frame #1 {
        n174 = call <instrlib>:"niDMM Read.vi"("error in (no error)"=w387, "instrument handle"=w384) -> ("error out"=w381:errorcluster, "Measurement"=w377:dbl, "instrument handle out"=w382:refnum<k15>)  [unwired: 7 in]
        "Current, A" <- w377
        n175 = Fract/Exp String To Number(string="NI DMM 1 units 3") -> (number=w385:dbl)  [unwired: 3 in, 1 out]
        n176 = Multiply(x=w385, y=w377) -> (x*y=w378:dbl)
        n177 = Absolute Value(x=w378) -> (abs(x)=→"Current Char":dbl)
        n178 = Absolute Value(x=w378) -> (abs(x)=→"Current":dbl)
        n179 = local read "Стоп"() -> (w383:bool)
      }
    }
    n180 = call <vilib>:"Simple Error Handler.vi"("error in (no error)"=w361) -> ("error out"=w366:errorcluster)  [unwired: 1 in, 7 out]
  }
  n181 = while {
    tunnel: w2 -> [w389]
    tunnel: w5 -> [w391]
    tunnel: [w389] -> w9
    tunnel: w3 -> [w392]
    stop <- w388 stop-if-true
    # "Управление шаговым двигателем"
    n182 = Wait (ms)(milliseconds to wait=u32 1) -> ()  [unwired: 1 out]
    n183 = event shown="[0] \"Погнали!\": Value Change" {
      selector: _ -> [_ _ _]
      dyn-events: _ -> [_ _ _]
      timeout: _ -> [_ _ _]
      tunnel: w389 -> [w397 w425 _]
      tunnel: w392 -> [w396 _ _]
      tunnel: w391 -> [w395 _ _]
      tunnel: [_ _ w431] -> w388
      event "Погнали!": Value Change {
        n184 = event-data() -> ("NewVal"=w393:bool)  [unwired: 1 in, 5 out]
        n185 = case shown="True" w393 {
          tunnel: "Go To" -> [_ w401]
          tunnel: w397 -> [_ w400]
          tunnel: w396 -> [_ _]
          tunnel: w395 -> [_ w399]
          frame False {
            n186 = Wait (ms)(milliseconds to wait=u32 1) -> ()  [unwired: 1 out]
          }
          frame True {
            n187 = while {
              tunnel: w401 -> [w408]
              tunnel: w400 -> [w409]
              tunnel: w399 -> [w411]
              stop <- w412 stop-if-true
              n188 = invoke class="AmateurStepperMotor" method="GoTo"(reference=w409, "destinationPosition"=w408) -> (reference out=w404:refnum<k24>, "GoTo"=w407:refnum<k24>)  [unwired: 2 in, 2 out]
              n189 = invoke class="Task" method="ConfigureAwait"(reference=w407, "continueOnCapturedContext"=FALSE) -> ()  [unwired: 2 in, 4 out]
              n190 = Wait (ms)(milliseconds to wait=u32 1) -> ()  [unwired: 1 out]
              n191 = while {
                tunnel: [w413] -> _
                tunnel: [w415] -> w405
                tunnel: [w417] -> w412
                tunnel: w408 -> [w422]
                tunnel: w411 -> [w420]
                tunnel: w404 -> [w414]
                stop <- w417 stop-if-true
                n192 = property class="AmateurStepperMotor"(reference=w414) -> (reference out=w415:refnum<k24>, "Position"=w413:dbl)  [unwired: 1 in, 1 out]
                "Position" <- w413
                n193 = Subtract(x=w413, y=w422) -> (x-y=w423:dbl)
                n194 = Wait (ms)(milliseconds to wait=u32 1) -> ()  [unwired: 1 out]
                n195 = Absolute Value(x=w423) -> (abs(x)=w421:dbl)
                n196 = Less Or Equal?(x=w421, y=w420) -> (x <= y?=w419:bool)
                n197 = Or(x=w419, y="Стоп GoTo") -> (x .or. y?=w417:bool)
                "Готово" <- w417
              }
              n198 = invoke class="AmateurStepperMotor" method="Stop"(reference=w405) -> (reference out=w403:refnum<k24>)  [unwired: 2 in, 2 out]
              n199 = property class="AmateurStepperMotor"(reference=w403) -> ("Position"=w402:dbl)  [unwired: 1 in, 2 out]
              n200 = local write "Position"(w402) -> ()
            }
          }
        }
      }
      event "set pos": Value Change {
        n201 = event-data() -> ("NewVal"=w426:bool)  [unwired: 1 in, 5 out]
        n202 = case shown="False" w426 {
          tunnel: w425 -> [_ w430]
          tunnel: "new pos" -> [_ w429]
          frame False {
          }
          frame True {
            n203 = property class="AmateurStepperMotor"(reference=w430, "Position"=w429) -> (reference out=w428:refnum<k24>)  [unwired: 1 in, 1 out]
            n204 = property class="AmateurStepperMotor"(reference=w428) -> ("Position"=w427:dbl)  [unwired: 1 in, 2 out]
            n205 = local write "Position"(w427) -> ()
          }
        }
      }
      event "Стоп": Value Change {
        n206 = event-data() -> ()  [unwired: 1 in, 6 out]
        n207 = local read "Стоп"() -> (w431:bool)
      }
    }
  }
  n208 = while {
    shift-right: [w434] -> _
    shift-left: 0 -> [w435]
    tunnel: w41 -> [_]
    stop <- w438 stop-if-true
    # "Управление Ардуино тумблерами"
    n209 = local read "Стоп"() -> (w438:bool)
    n210 = Wait (ms)(milliseconds to wait=u32 10 ("millisecond timer value")) -> ()  [unwired: 1 out]
    n211 = Boolean Array To Number(Boolean array="Сегменты") -> (number=w433:u32)
    n212 = To Long Integer(number=w433) -> (32bit integer=w434:i32)
    n213 = Not Equal?(x=w434, y=w435) -> (x != y?=w436:bool)
    n214 = case shown="True" w436 {
      tunnel: w434 -> [_ w439]
      tunnel: w435 -> [_ w440]
      frame False {
      }
      frame True {
        n215 = stacked-sequence {
          seq-local: [w443 _ _] -> [_ w454 _]
          seq-local: [w441 _ _] -> [_ w449 _]
          seq-local: [_ w450 _] -> [_ _ w490]
          tunnel: w439 -> [w445 _ _]
          tunnel: w440 -> [w444 _ _]
          frame #0 {
            # "Детектирвоание позиции и\nнаправления изменения бита"
            n216 = Subtract(x=w445, y=w444) -> (x-y=w446:i32)
            n217 = To Double Precision Float(number=w446) -> (double precision float=w447:dbl)
            n218 = Greater Than 0?(x=w446) -> (x > 0?=w443:bool)
            "+/-" <- w443
            n219 = Absolute Value(x=w447) -> (abs(x)=w442:dbl)
            n220 = Logarithm Base 2(1:w442) -> (0:w441:dbl)
            "Разряд" <- w441
          }
          frame #1 {
            # "Указывает на последнюю нажатую кнопку"
            # "Выбор бита и направления\n его измнения"
            n221 = case shown="10" w449 {
              tunnel: ["D10" "D9" "D5" "D8" "D11" "D12" "A1" "D4" "A5" "A4" "A3" "A2" "A0" "D13" "D3" "All"] -> w452
              tunnel: ["a" "b" "c" "d" "e" "f" "g" "h" "j" "k" "L" "m" "n" "p" "dp" "All"] -> w448
              frame 0, Default {
                # "a = D10"
              }
              frame 1 {
                # "b = D9"
              }
              frame 2 {
                # "c = D5"
              }
              frame 3 {
                # "d = D8"
              }
              frame 4 {
                # "e = D11"
              }
              frame 5 {
                # "f = D12"
              }
              frame 6 {
                # "g = A1"
              }
              frame 7 {
                # "h = D4"
              }
              frame 8 {
                # "j = A5"
              }
              frame 9 {
                # "k = A4"
              }
              frame 10 {
                # "L = A3"
              }
              frame 11 {
                # "m = A2"
              }
              frame 12 {
                # "n = A0"
              }
              frame 13 {
                # "p = D13"
              }
              frame 14 {
                # "dp = D3"
              }
              frame 15 {
              }
            }
            "Сегмент" <- w448
            n222 = Select(t="off", s=w454, f="on") -> (s? t:f=w451:string)
            n223 = Concatenate Strings(w452, "_" ("string"), w451) -> (w450:string)
          }
          frame #2 {
            # "Передача команды в Ардуино"
            n224 = Equal?(x=w490, y="All_off") -> (x = y?=w493:bool)
            n225 = Equal?(x=w490, y="All_on") -> (x = y?=w491:bool)
            n226 = case shown="True" w493 {
              frame False {
              }
              frame True {
                n227 = local write "Сегменты"(bool[] [TRUE, TRUE, TRUE, TRUE, TRUE, TRUE, TRUE, TRUE, TRUE, TRUE, TRUE, TRUE, TRUE, TRUE, TRUE, TRUE] ("Сегменты")) -> ()
              }
            }
            n228 = case shown="True" w491 {
              frame False {
              }
              frame True {
                n229 = local write "Сегменты"(bool[] [FALSE, FALSE, FALSE, FALSE, FALSE, FALSE, FALSE, FALSE, FALSE, FALSE, FALSE, FALSE, FALSE, FALSE, FALSE, FALSE] ("Сегменты")) -> ()
              }
            }
            n230 = stacked-sequence {
              tunnel: w490 -> [w496 _ _]
              frame #0 {
                n231 = local write "Command"(w496) -> ()
              }
              frame #1 {
                n232 = local write "Записать"(TRUE ("Записать")) -> ()
                n233 = Wait (ms)(milliseconds to wait=u32 1000) -> ()  [unwired: 1 out]
              }
              frame #2 {
                n234 = local write "Записать"(FALSE ("Записать")) -> ()
                n235 = Wait (ms)(milliseconds to wait=u32 1000) -> ()  [unwired: 1 out]
              }
            }
          }
        }
      }
    }
  }
  n236 = call <instrlib>:"niDMM Close.vi"("error in (no error)"=w34, "instrument handle"=w35) -> ()  [unwired: 9 in, 1 out]
  n237 = while {
    tunnel: [w507] -> w36
    tunnel: w39 -> [w505]
    tunnel: w38 -> [w504]
    tunnel: [w501] -> w37
    stop <- w503 stop-if-true
    # "Настройка вольтметра NI PXI-4071"
    n238 = Wait (ms)(milliseconds to wait=u32 1) -> ()  [unwired: 1 out]
    n239 = flat-sequence {
      tunnel: [w514] -> w509
      tunnel: w505 -> [w512]
      tunnel: w504 -> [w516]
      tunnel: [w513] -> w508
      tunnel: w509 -> [w525]
      tunnel: w508 -> [w528]
      tunnel: [w524] -> w503
      tunnel: [w523] -> w501
      tunnel: [w522] -> w502
      frame #0 {
        w510 = T6 6.5 items=["3 1/2"=3.5, "4 1/2"=4.5, "5 1/2"=5.5, "6 1/2"=6.5, "7 1/2"=7.5] ("Resolution in Digits")
        n240 = Fract/Exp String To Number(string="NI DMM 1 Voltage Range 4") -> (number=w515:dbl)  [unwired: 3 in, 1 out]
        n241 = call-poly <instrlib>:"niDMM Config Measurement.vi"("Range"=w515, "Resolution in Digits"=w510, "error in (no error)"=w516, "Function"=niDMM_Function."DC Volts" ("Measurement Type"), "instrument handle"=w512) -> ("error out"=w513:errorcluster, "instrument handle out"=w514:refnum<k15>)  [unwired: 5 in]
      }
      frame #1 {
        n242 = call <instrlib>:"niDMM Read.vi"("error in (no error)"=w528, "instrument handle"=w525) -> ("error out"=w522:errorcluster, "Measurement"=w520:dbl, "instrument handle out"=w523:refnum<k15>)  [unwired: 7 in]
        "Voltage, V" <- w520
        n243 = Fract/Exp String To Number(string="NI DMM 1 units 4") -> (number=w526:dbl)  [unwired: 3 in, 1 out]
        n244 = Multiply(x=w526, y=w520) -> (x*y=w518:dbl)
        n245 = Absolute Value(x=w518) -> (abs(x)=→"Voltage Char":dbl)
        n246 = Absolute Value(x=w518) -> (abs(x)=→"Voltage":dbl)
        n247 = local read "Стоп"() -> (w524:bool)
      }
    }
    n248 = call <vilib>:"Simple Error Handler.vi"("error in (no error)"=w502) -> ("error out"=w507:errorcluster)  [unwired: 1 in, 7 out]
  }
  n249 = invoke class="AmateurStepperMotor" method="Stop"(reference=w9) -> (reference out=w16:refnum<k24>, "Stop"=w17:refnum<k24>)  [unwired: 2 in, 1 out]
  n250 = property class="AmateurStepperMotor"(reference=w16, "HoldOn"=FALSE) -> (reference out=w15:refnum<k24>)  [unwired: 1 in, 1 out]
  n251 = invoke class="AmateurStepperMotor" method="Dispose"(reference=w15) -> (error out=w12:errorcluster)  [unwired: 2 in, 2 out]
  n252 = invoke class="SerialPort" method="Close"(reference=w27, error in=w12) -> (reference out=w11:refnum<k24>, error out=w13:errorcluster)  [unwired: 1 in, 1 out]
  n253 = invoke class="Task" method="Wait"(reference=w17) -> ()  [unwired: 2 in, 3 out]
  n254 = Close Reference(reference=w11, error in (no error)=w13) -> (error out=w14:errorcluster)
  n255 = call <vilib>:"Simple Error Handler.vi"("error in (no error)"=w14) -> ()  [unwired: 1 in, 8 out]
  n256 = VISA Close(VISA resource name=w20, error in (no error)=w19) -> (error out=w29:errorcluster)
  n257 = call <instrlib>:"niDMM Close.vi"("error in (no error)"=w36, "instrument handle"=w37) -> ()  [unwired: 9 in, 1 out]
  n258 = call <instrlib>:"niDCPower Close.vi"("instrument handle"=w42) -> ()  [unwired: 10 in, 1 out]
  n259 = call "Ophir Error Message.vi"("error in (no error)"=w29) -> ()  [unwired: 3 in, 4 out]
  n260 = disable-structure shown="Disabled" {
    frame Disabled {
    }
    frame Enabled {
    }
  }
